vi "DHA Desnsity of Humid Air(kg to m3).vi"(1 "Total Pressure of Humid Air":dbl[unit], 2 "Tceg":dbl[unit], 3 "RH":dbl) -> (0 "DHA":dbl[unit])   [LabVIEW 2018]
panel:
  out "DHA\nDesnsity of Humid Air\nDHA=PDWV+PDDA":dbl[unit](knob) scale=0.0..1.0
  out "Temprature Of Input Air\nKelvin Degree":dbl[unit](slide) scale=273.0..373.0
  out "Tk":dbl[unit]
  out "Temprature Of Input Air\nCentigrade Degree":dbl[unit](slide) scale=0.0..100.0
  out "Humidity of Input Air":dbl(knob) scale=0.0..100.0
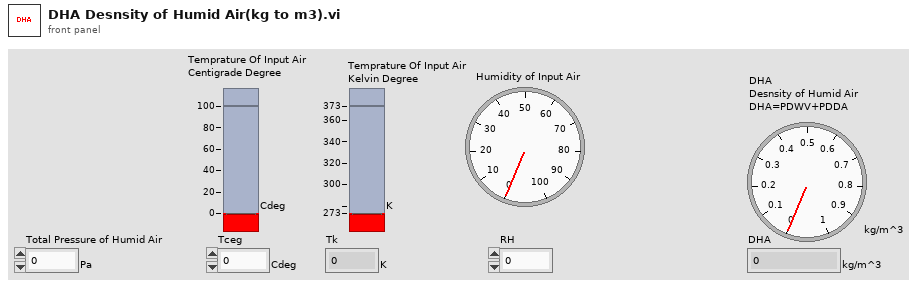
[diagram p1: front panel]
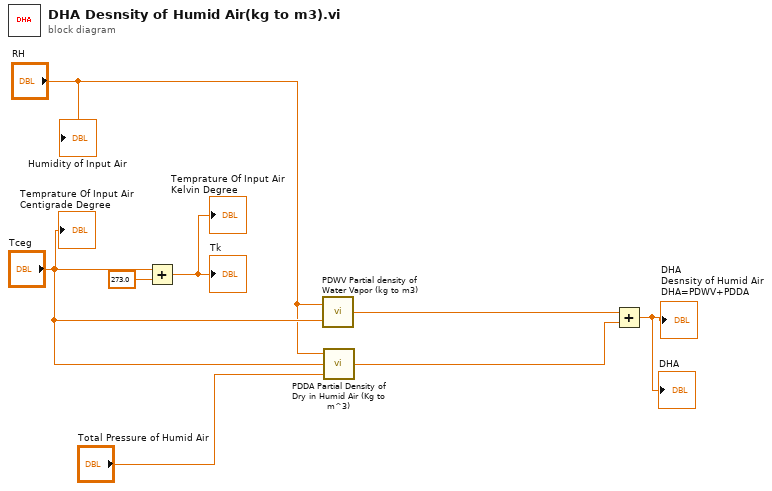
[diagram p0: block diagram]
diagram:
  n1 = Add(x="Tceg", y=dbl[unit] 273.0) -> (x+y=→"Tk" →"Temprature Of Input Air\nKelvin Degree":dbl[unit])
  n2 = call "PDWV Partial density of Water Vapor (kg to m3).vi"("Tceg"="Tceg", "RH"="RH") -> ("PDWV"=w6:dbl[unit])
  n3 = call "PDDA Partial Density of Dry in Humid Air (Kg to m^3).vi"("Total Pressure of Humid Air"="Total Pressure of Humid Air", "Tceg"="Tceg", "RH"="RH") -> ("PDDA"=w4:dbl[unit])
  n4 = Add(x=w6, y=w4) -> (x+y=→"DHA\nDesnsity of Humid Air\nDHA=PDWV+PDDA" →"DHA":dbl[unit])
  "Humidity of Input Air" <- "RH"
  "Temprature Of Input Air\nCentigrade Degree" <- "Tceg"
